vi "Close.vi"(8 "error in (no error)":errorcluster, 11 "object in":refnum<class "TableLogger_CSV_Actor.lvclass">) -> (0 "error out":errorcluster, 3 "object out":refnum<class "TableLogger_CSV_Actor.lvclass">)   [LabVIEW 2014, in "TableLogger_CSV_Actor.lvlib" / "TableLogger_CSV_Actor.lvclass"]
uses:
  TableLogger_CSV_Actor.lvclass
  TableLogger_CSV_Actor.lvclass/TableLogger_CSV_Actor.ctl
panel:
  # "Connector Pane"
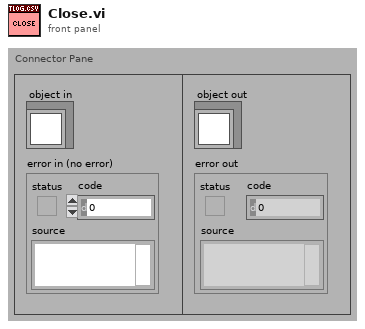
[diagram p1: front panel]
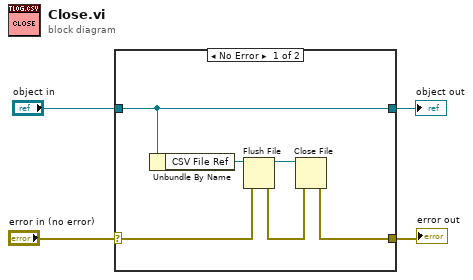
[diagram p0: block diagram]
diagram:
  n1 = case shown="No Error" "error in (no error)" {
    selector: "error in (no error)" -> [w10 w12]
    tunnel: [w8 w12] -> w3
    tunnel: [w9 w11] -> w1
    tunnel: "object in" -> [w9 w11]
    frame No Error {
      n2 = Unbundle By Name(w9) -> ("CSV File Ref"=w6:refnum<file>)
      n3 = Flush File(refnum=w6, error in=w10) -> (refnum out=w5:refnum<file>, error out=w7:errorcluster)
      n4 = Close File(refnum=w5, error in=w7) -> (error out=w8:errorcluster)  [unwired: 1 out]
    }
    frame Error {
    }
  }
  "error out" <- w3
  "object out" <- w1
